vi "receiveSerialNumber.vi"(8 "error in (no error)":errorcluster, 11 "TEI9150 in":refnum<class "TEI9150.lvclass">) -> (0 "error out":errorcluster, 2 "Serial Number":string, 3 "TEI9150 out":refnum<class "TEI9150.lvclass">)   [LabVIEW 2015, in "TEI9150.lvclass"]
uses:
  TEI9150.lvclass
  TEI9150.lvclass/TEI9150.ctl
  <userlib>/Common/SerialProtocols/SerialCommunicator/SerialCommunicator.lvclass
  <vilib>/regexp/Match Regular Expression.xnode
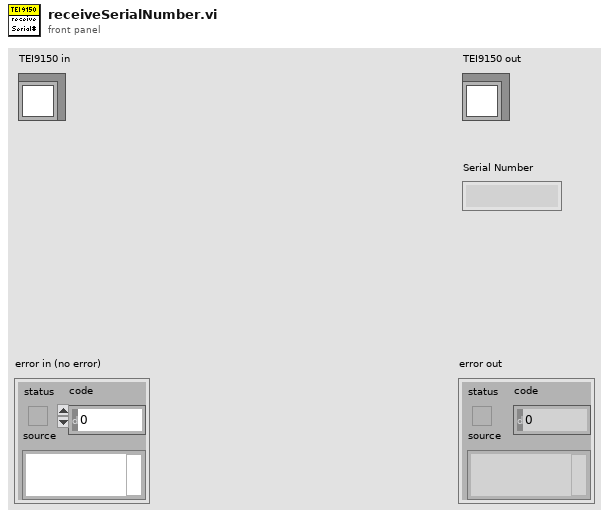
[diagram p1: front panel]
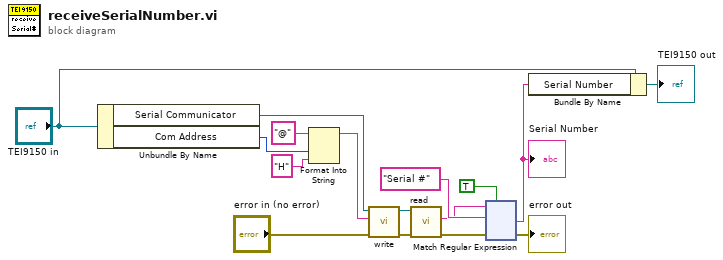
[diagram p0: block diagram]
diagram:
  n1 = Unbundle By Name("TEI9150 in") -> ("Serial Communicator"=w14:refnum<class "SerialCommunicator.lvclass">, "Com Address"=w12:u8)
  n2 = Format Into String(initial string="@" ("string"), w12, "H" ("string")) -> (resulting string=w10:string)  [unwired: 2 in, 1 out]
  n3 = call-dynamic "write.vi"("error in (no error)"="error in (no error)", "writeString"=w10, "SerialCommunicator in"=w14) -> ("error out"=w7:errorcluster, "SerialCommunicator out"=w9:refnum<class "SerialCommunicator.lvclass">)  [unwired: 7 in]
  n4 = call-dynamic "read.vi"("error in (no error)"=w7, "SerialCommunicator in"=w9) -> ("error out"=w5:errorcluster, "stringRead"=w6:string)  [unwired: 7 in, 1 out]
  n5 = xnode "Match Regular Expression"("input string"=w6, "regular expression"="Serial #", "error in"=w5, "ignore case? (F)"=TRUE) -> ("after match"=w3:string, "error out"=→"error out":errorcluster)  [unwired: 2 in, 3 out]
  "Serial Number" <- w3
  n6 = Bundle By Name(cluster="TEI9150 in", "Serial Number"=w3) -> (→"TEI9150 out":refnum<class "TEI9150.lvclass">)
